vi "LEBITplc.IGCalibration.vi"(0 "Enum":enum16{"DelayedDC", "MASSTOAMP", "AMPTOMASS"}(ring), 1 "i attribute":T1, 3 "MASS":dbl, 4 "AMP":dbl) -> (16 "Delayed DC":string[][](array[string]), 17 "AMP":dbl, 18 "MASS":dbl)   [LabVIEW 2014, in "LEBITplc.lvlib"]
uses:
  LEBITplc.lvlib
  LEBITplc.i attribute.ctl
  <vilib>/express/express arith-compare/Formula/XNode/ExpressFormulaBlockNode.xnode
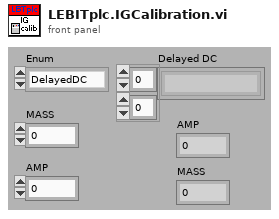
[diagram p1: front panel]
types:
  T1 = typedef "LEBITplc.lvlib/LEBITplc.i attribute.ctl" = cluster{"LLFLocation":string, "SetFileLocation":string, "nickNames":string[], "setValuePLCServiceID":i32[], "GUIServiceID":i32[], "monValuePLC":string[], "SetValueServiceID":i32[], "MonValueServiceID":i32[], "SetValue":dbl[][], "SetValueMin":dbl[], "SetValueMax":dbl[], "SetValueInfoServiceID":i32[], "GUINames":string[], "ListOfBases":string[], "Scale":dbl[], "Offset":dbl[], "setValuePLC":string[], "BaseName":string[], "ScaleServiceID":i32[], "OffsetServiceID":i32[], "AllPLCValues":string[], "CondSpecialArray":string[][], "CondSpecialIndex":i32[], "CondSpecialMonValue":dbl[], "RecentlyChanged":i32[], "SetFileLocationID":i32, "Dependent-Monitors":string[][], "LastLoadedFiles":string[], "IonGuideCalibLocation":string, "Monitor Dependent":string[], "Special":string[], "PLC?":bool[], "Start Date":string, "ListOfBasesServiceID":i32, "SETRA VISA resource":refnum<visa-resource-name>}
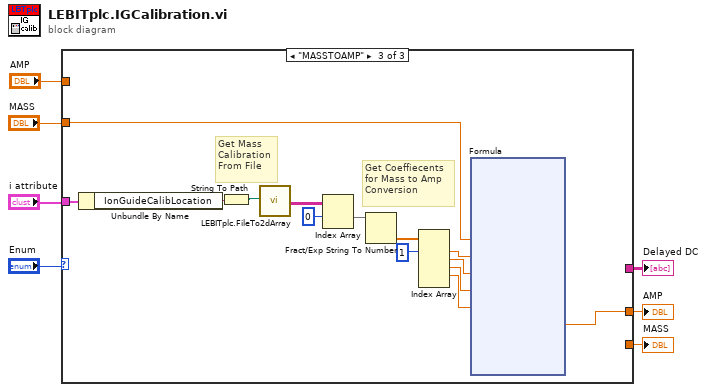
[diagram p0: block diagram]
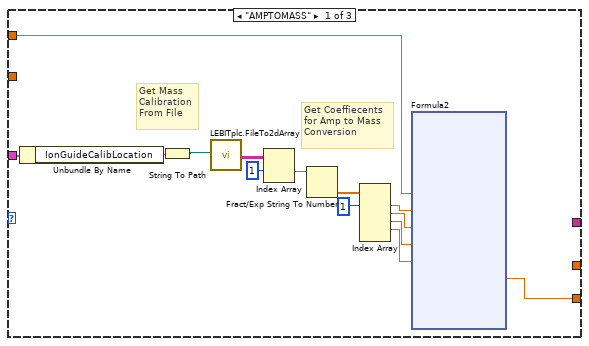
[diagram p2: hidden frame]
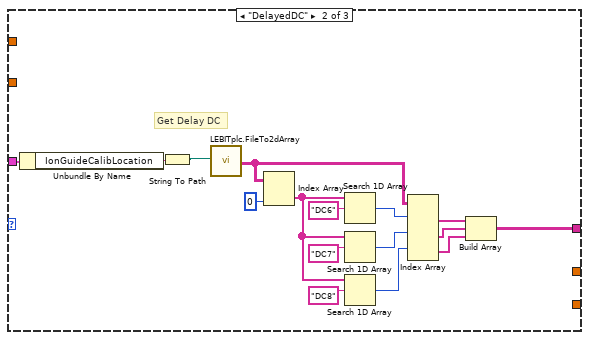
[diagram p3: hidden frame]
diagram:
  n1 = case shown="\"MASSTOAMP\"" "Enum" {
    tunnel: "MASS" -> [_ _ w59]
    tunnel: "i attribute" -> [w9 w51 w56]
    tunnel: [_ _ w54] -> w4
    tunnel: "AMP" -> [w10 _ _]
    tunnel: [w8 _ _] -> w2
    tunnel: [_ w38 _] -> w1
    frame "AMPTOMASS" {
      # "Get Coeffiecents\nfor Amp to Mass\nConversion"
      # "Get Mass \nCalibration\nFrom File"
      n2 = Unbundle By Name(w9) -> ("IonGuideCalibLocation"=w12:string)
      n3 = String To Path(string=w12) -> (path=w13:path)
      n4 = call "LEBITplc.FileTo2dArray.vi"("file path (dialog if empty)"=w13) -> ("Array"=w21:string[][])  [unwired: 17 in, 1 out]
      n5 = Index Array(array=w21, index (row)=1) -> (element=w19:string[])  [unwired: 1 in]
      n6 = Fract/Exp String To Number(string=w19) -> (number=w18:dbl[])  [unwired: 3 in, 1 out]
      n7 = Index Array(array=w18, index #1=1 ("index")) -> (element #1=w17:dbl, element #2=w16:dbl, element #3=w15:dbl, element #4=w14:dbl)  [unwired: 4 in, 1 out]
      n8 = xnode "Formula2"("X"=w10, "a0"=w17, "a1"=w16, "a2"=w15, "a3"=w14) -> ("Result"=w8:dbl)  [unwired: 1 in, 1 out]
    }
    frame "DelayedDC" {
      # "Get Delay DC"
      n9 = Unbundle By Name(w51) -> ("IonGuideCalibLocation"=w52:string)
      n10 = String To Path(string=w52) -> (path=w53:path)
      n11 = call "LEBITplc.FileTo2dArray.vi"("file path (dialog if empty)"=w53) -> ("Array"=w44:string[][])  [unwired: 17 in, 1 out]
      n12 = Index Array(array=w44, index (col)=0 ("index (row)")) -> (element=w49:string[])  [unwired: 1 in]
      n13 = Search 1D Array(1D array=w49, element="DC6") -> (index of element=w45:i32)  [unwired: 1 in]
      n14 = Search 1D Array(1D array=w49, element="DC7") -> (index of element=w43:i32)  [unwired: 1 in]
      n15 = Search 1D Array(1D array=w49, element="DC8") -> (index of element=w42:i32)  [unwired: 1 in]
      n16 = Index Array(array=w44, index (row) #1=w45, index (row) #2=w43, index (row) #3=w42) -> (element #1=w41:string[], element #2=w40:string[], element #3=w39:string[])  [unwired: 3 in]
      n17 = Build Array(w41, w40, w39) -> (w38:string[][])
    }
    frame "MASSTOAMP" {
      # "Get Coeffiecents\nfor Mass to Amp\nConversion"
      # "Get Mass \nCalibration\nFrom File"
      n18 = Unbundle By Name(w56) -> ("IonGuideCalibLocation"=w57:string)
      n19 = String To Path(string=w57) -> (path=w58:path)
      n20 = call "LEBITplc.FileTo2dArray.vi"("file path (dialog if empty)"=w58) -> ("Array"=w67:string[][])  [unwired: 17 in, 1 out]
      n21 = Index Array(array=w67, index (row)=0) -> (element=w65:string[])  [unwired: 1 in]
      n22 = Fract/Exp String To Number(string=w65) -> (number=w64:dbl[])  [unwired: 3 in, 1 out]
      n23 = Index Array(array=w64, index #1=1 ("index")) -> (element #1=w63:dbl, element #2=w62:dbl, element #3=w61:dbl, element #4=w60:dbl)  [unwired: 4 in, 1 out]
      n24 = xnode "Formula"("X"=w59, "a0"=w63, "a1"=w62, "a2"=w61, "a3"=w60) -> ("Result"=w54:dbl)  [unwired: 1 in, 1 out]
    }
  }
  "AMP" <- w4
  "MASS" <- w2
  "Delayed DC" <- w1
